vi "JKISM++ State Dashboard - DebugTool.vi"() -> ()   [LabVIEW 2014]
uses:
  _Support/Typedef/_JKI StateMachine Current State.ctl
  <resource>/dialog/lvconfig.llb/LV Config Read String.vi
  <resource>/dialog/lvconfig.llb/LV Config Read Numeric (I32).vi
  <resource>/dialog/lvconfig.llb/LV Config Write Numeric (I32).vi
  _Support/GlobalEvent/FGV-GlobalEventRef.vi
  _Support/jkism-tool-support.lvlib
  JKI-State-Machine-Plus.lvlib
panel:
  out "Dashboard":T1(array[cluster])
  out "State History":string
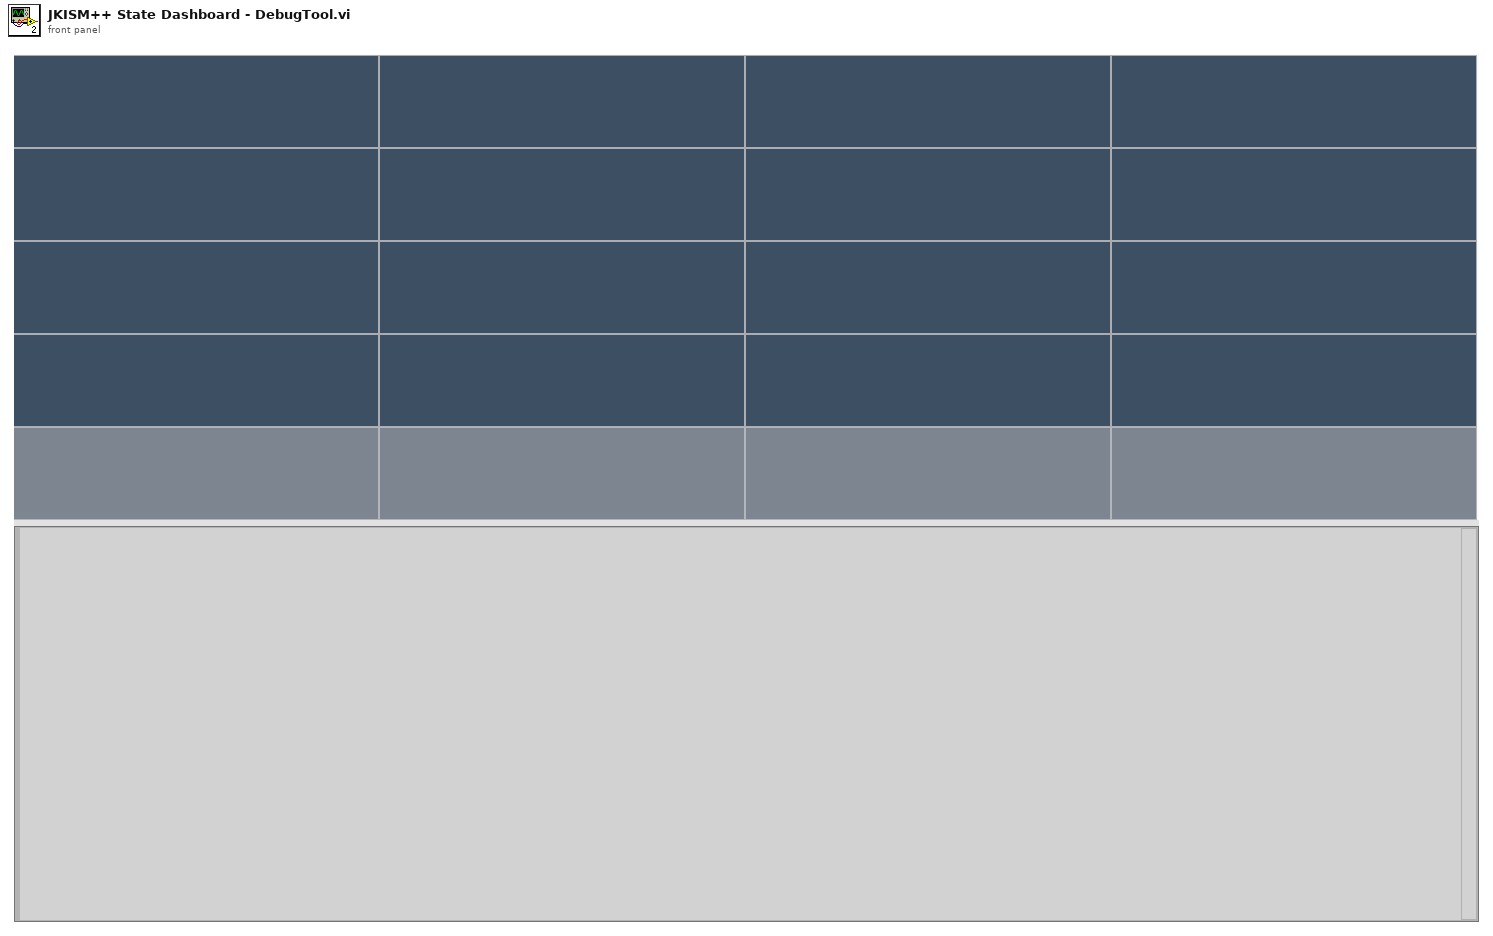
[diagram p1: front panel]
types:
  T1 = cluster{"Label":string, "Value":string, "String":string}[][]
  T2 = typedef "JKI-State-Machine-Plus.lvlib/_JKI StateMachine Current State.ctl" = cluster{"Name(\"\" to use uuid)":string, "Current State":string, "Arguments":string, "Argument - State":string, "From Who":string}
  T3 = enum32{"Invalid", "Standard", "Closed", "Hidden", "Minimized", "Maximized"}
  T4 = enum32{"invalid app kind", "Development System", "Run Time System", "Student Edition", "Embedded LabVIEW", "Evaluation", "Custom"}
  T5 = cluster{"Label":string, "Value":string, "String":string}
  T6 = cluster{"Core":cluster{"Current VI Reference":refnum<vi>, "Close Panel on Exit?":bool}, "Global-DataTable":string[][], "NumCols":i16, "NumRows":i16, "ApplicationName":string, "JKISM Global Log Event":refnum<user-event>}
  T7 = cluster{"Current VI Reference":refnum<vi>, "Close Panel on Exit?":bool}
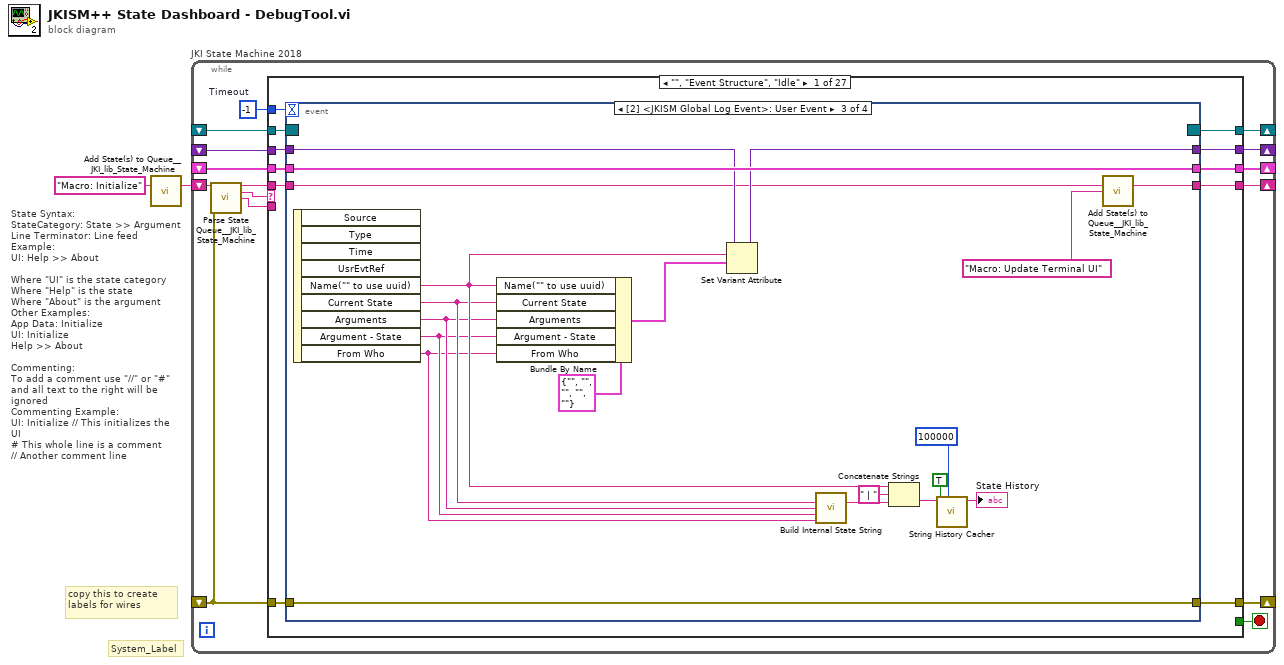
[diagram p0: block diagram]
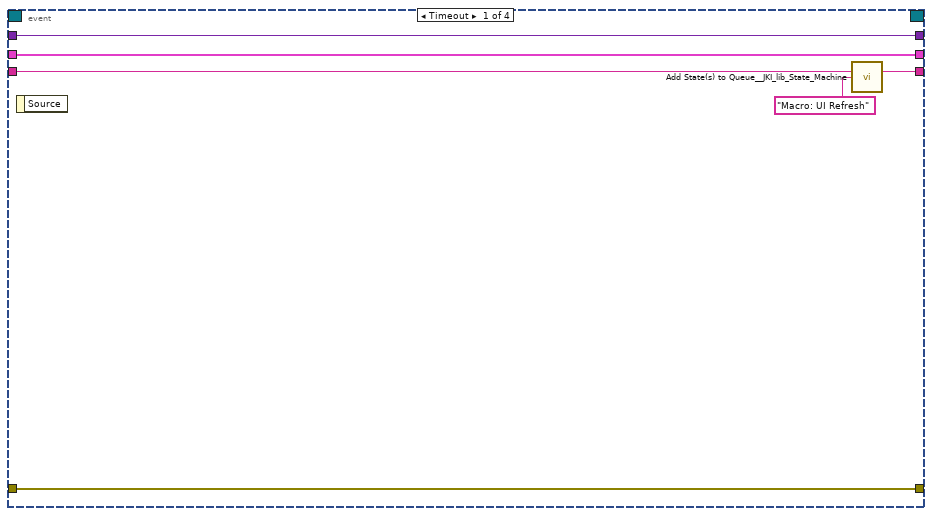
[diagram p2: hidden frame]
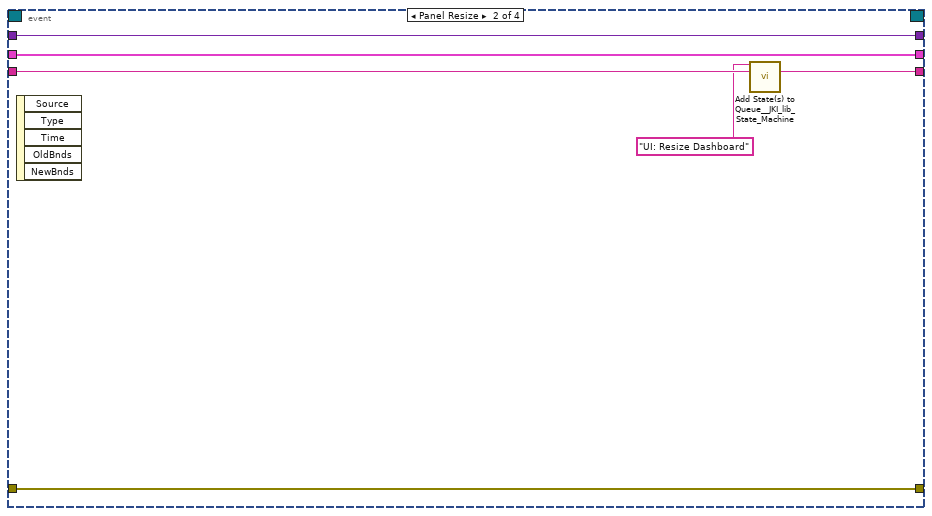
[diagram p3: hidden frame]
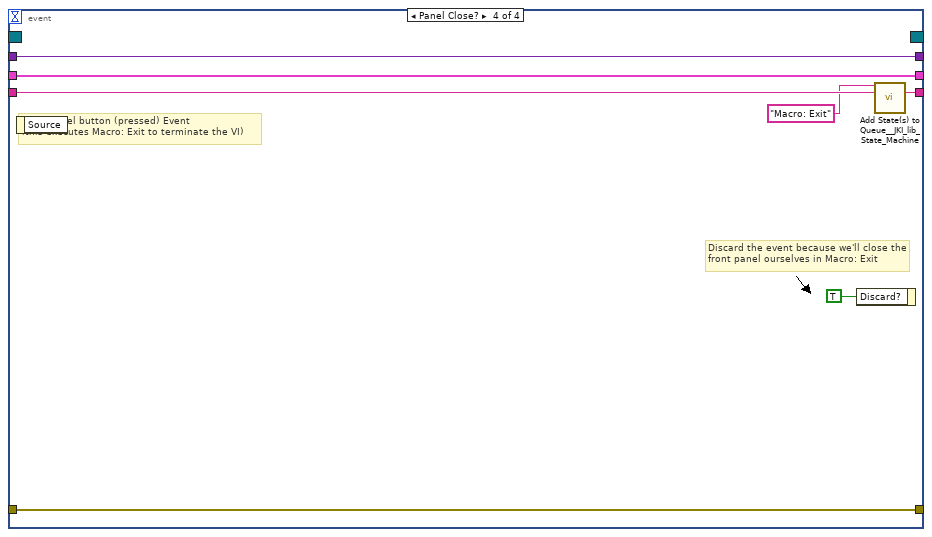
[diagram p4: hidden frame]
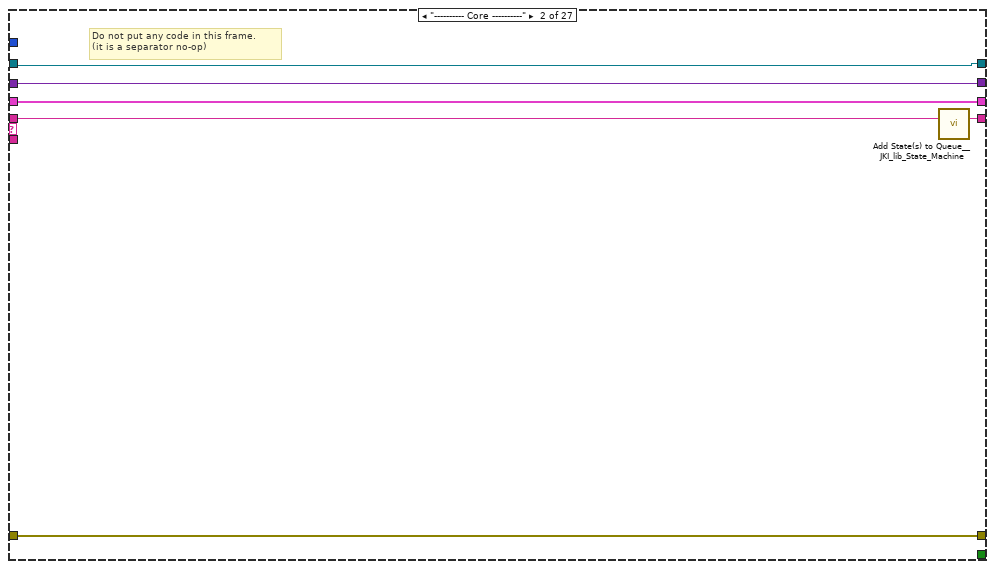
[diagram p5: hidden frame]
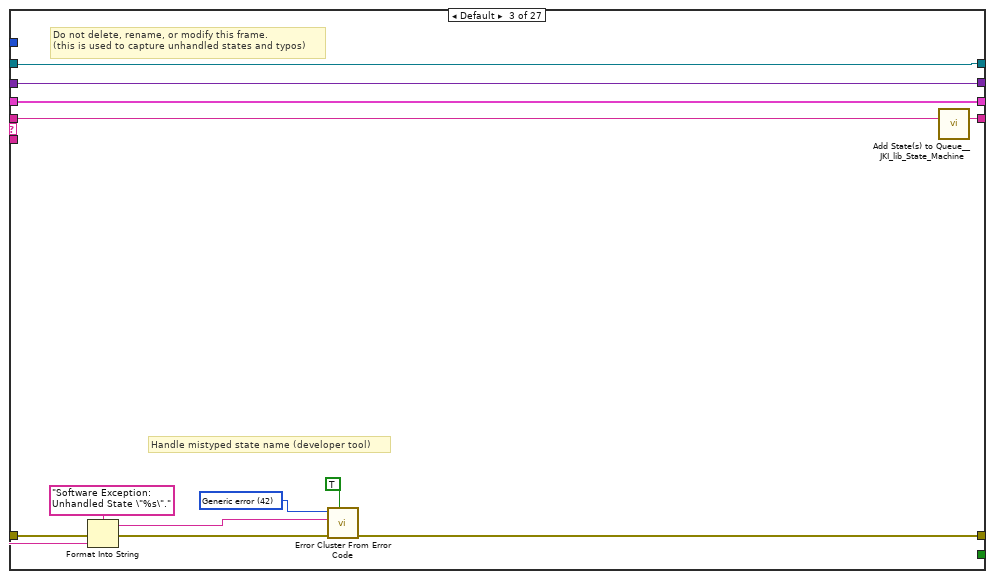
[diagram p6: hidden frame]
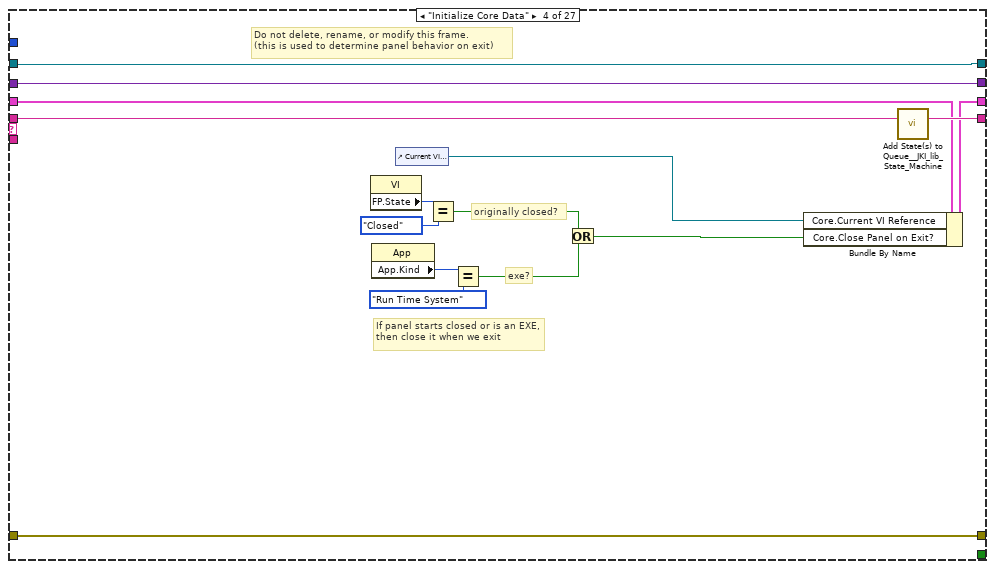
[diagram p7: hidden frame]
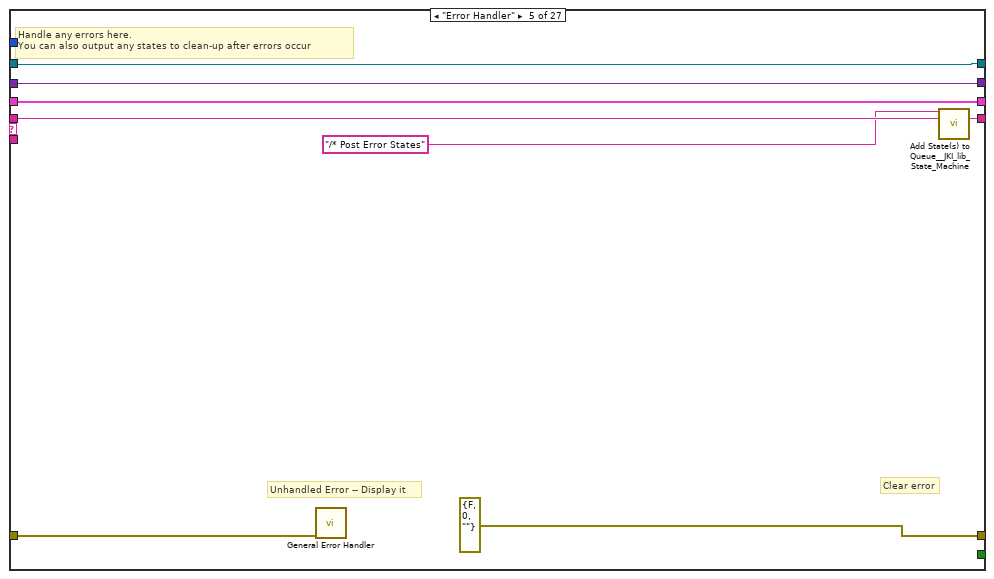
[diagram p8: hidden frame]
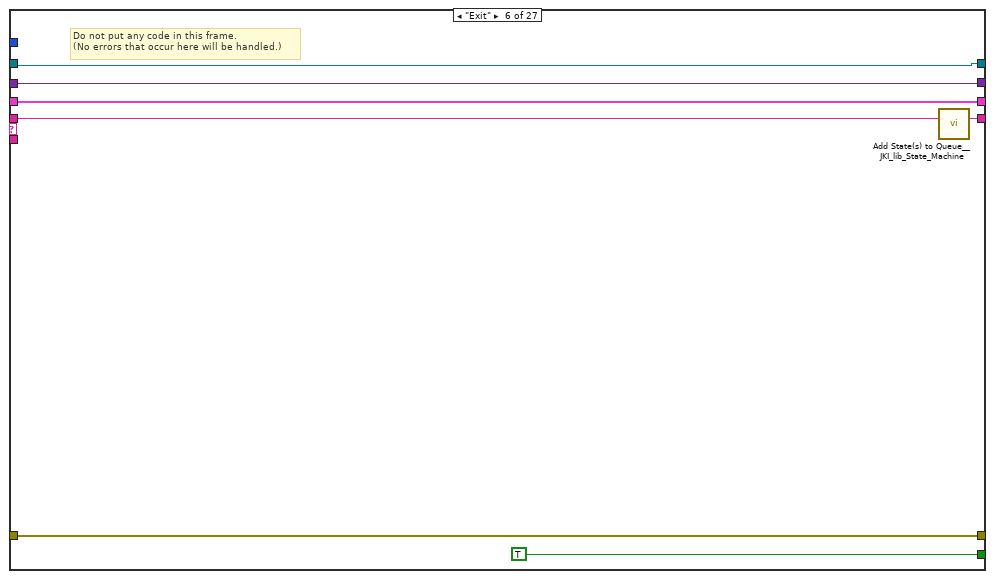
[diagram p9: hidden frame]
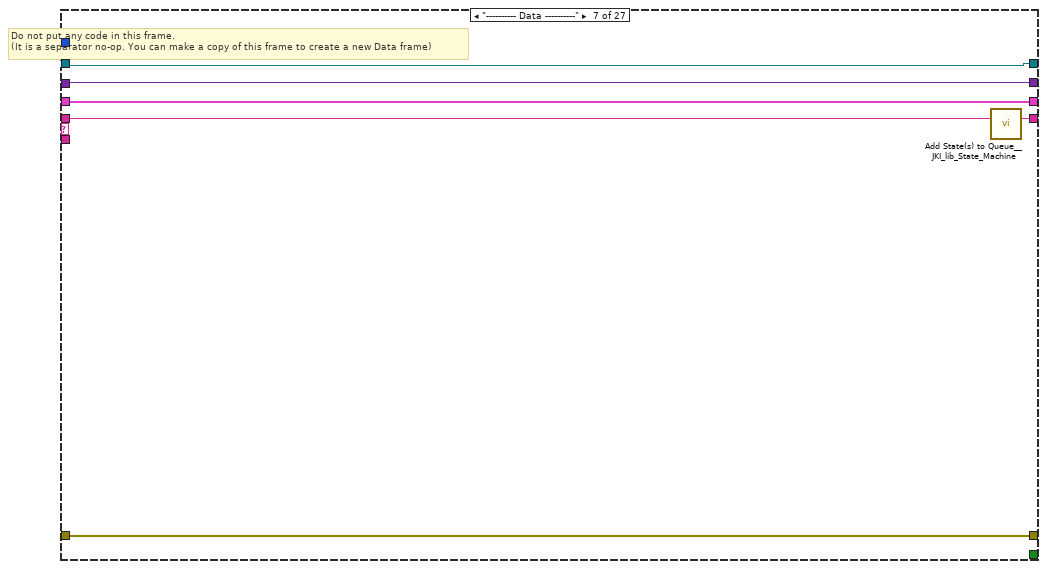
[diagram p10: hidden frame]
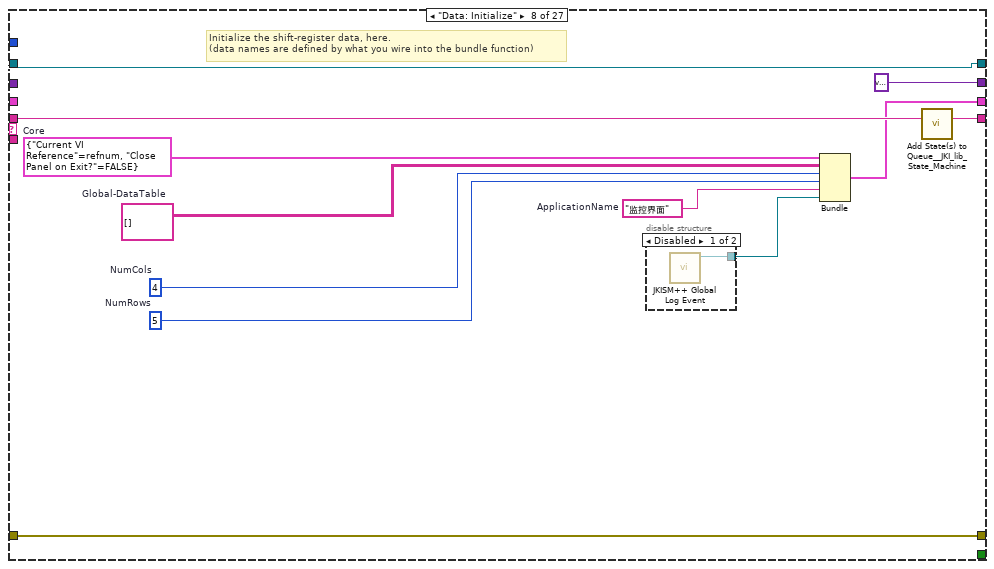
[diagram p11: hidden frame]
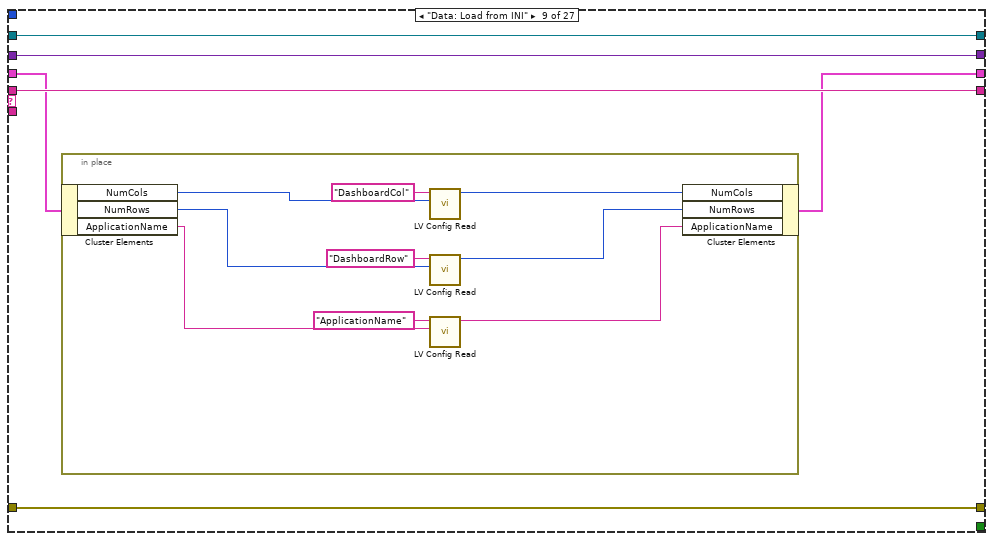
[diagram p13: hidden frame]
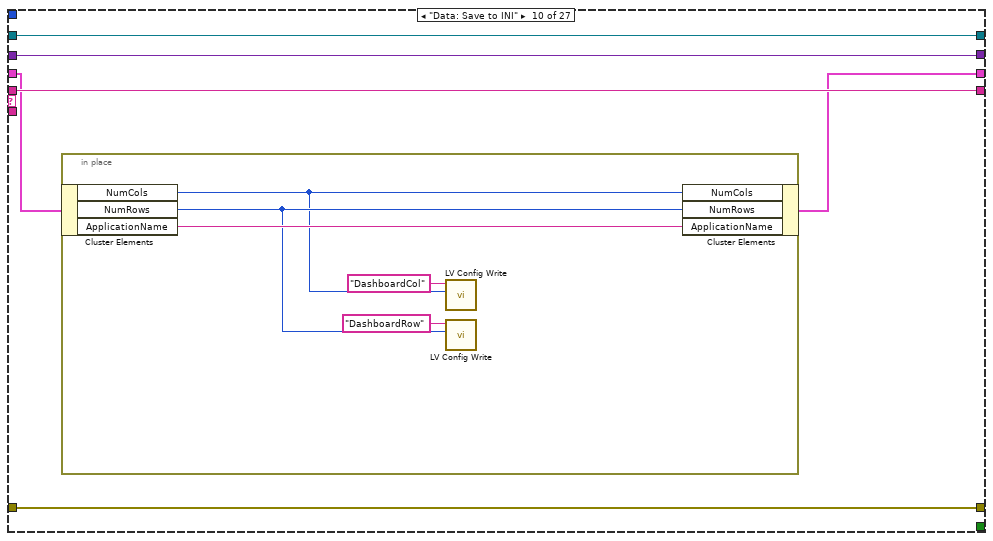
[diagram p14: hidden frame]
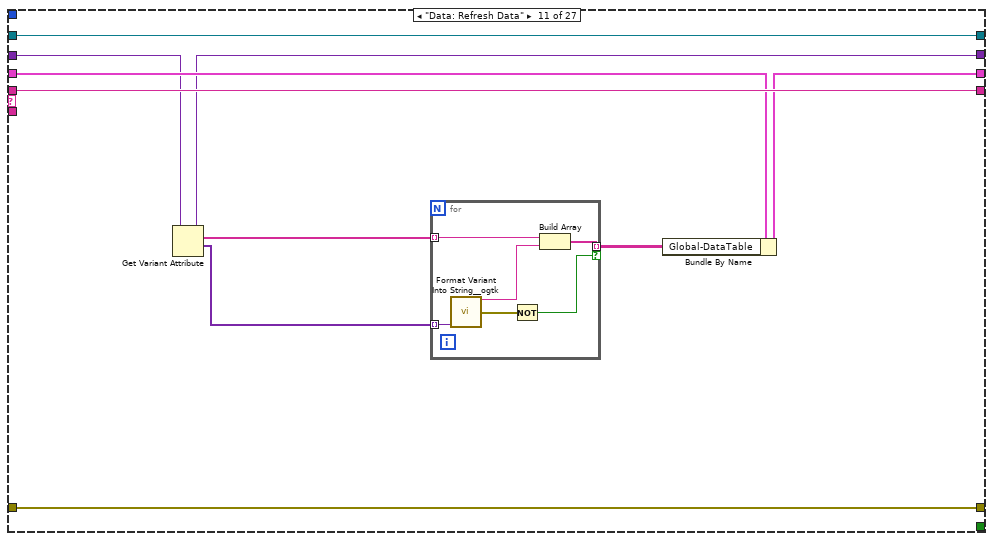
[diagram p15: hidden frame]
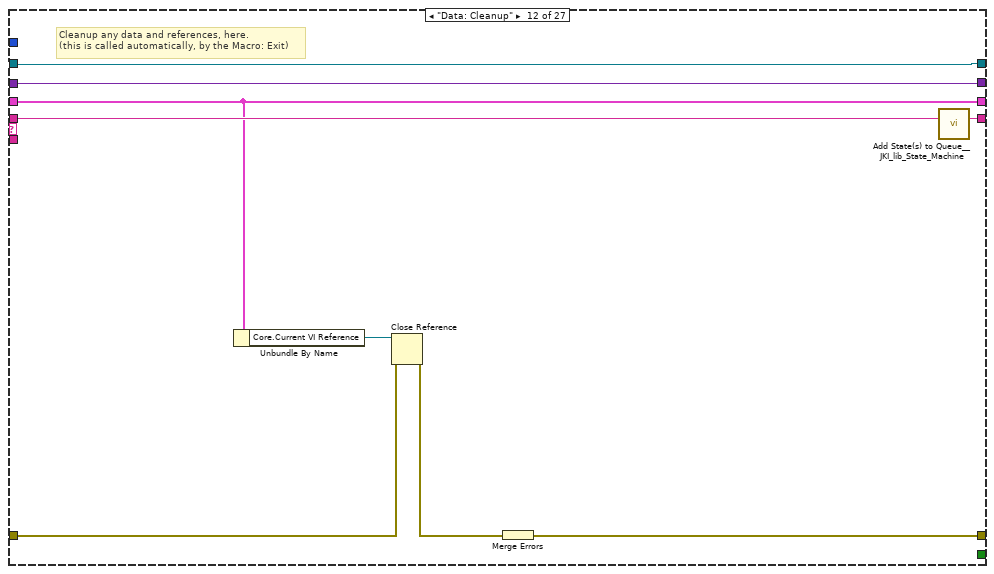
[diagram p16: hidden frame]
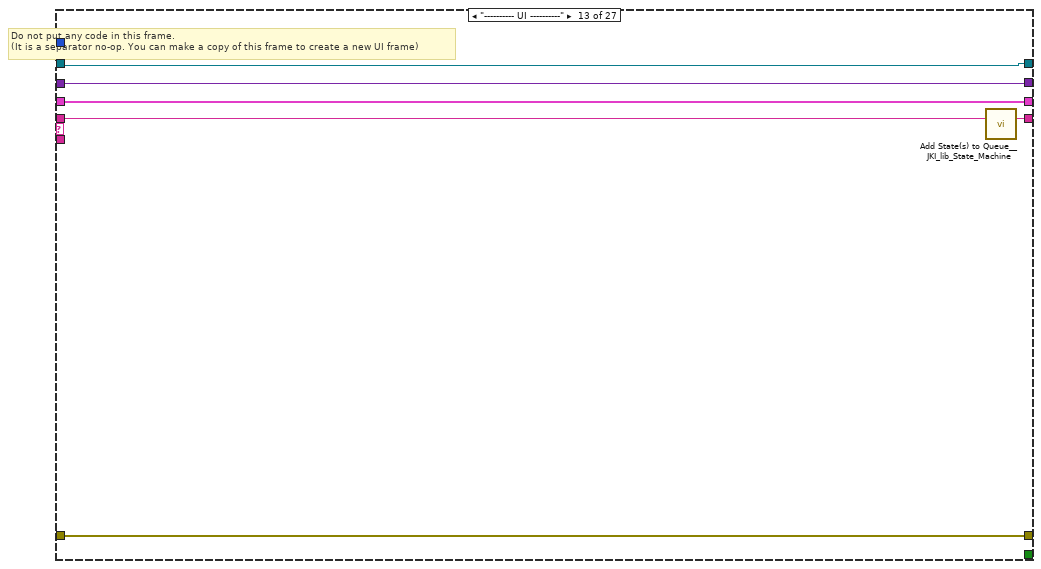
[diagram p17: hidden frame]
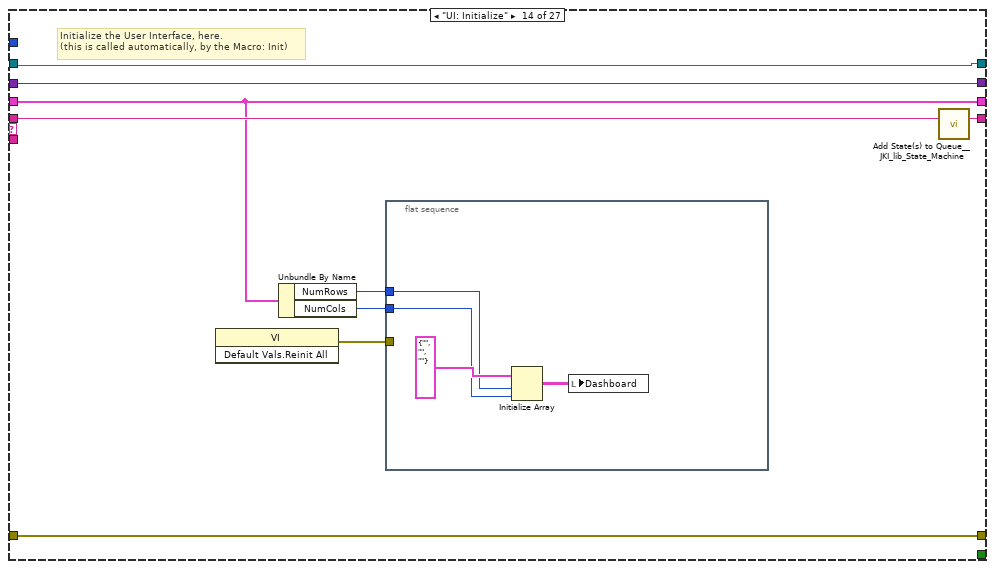
[diagram p18: hidden frame]
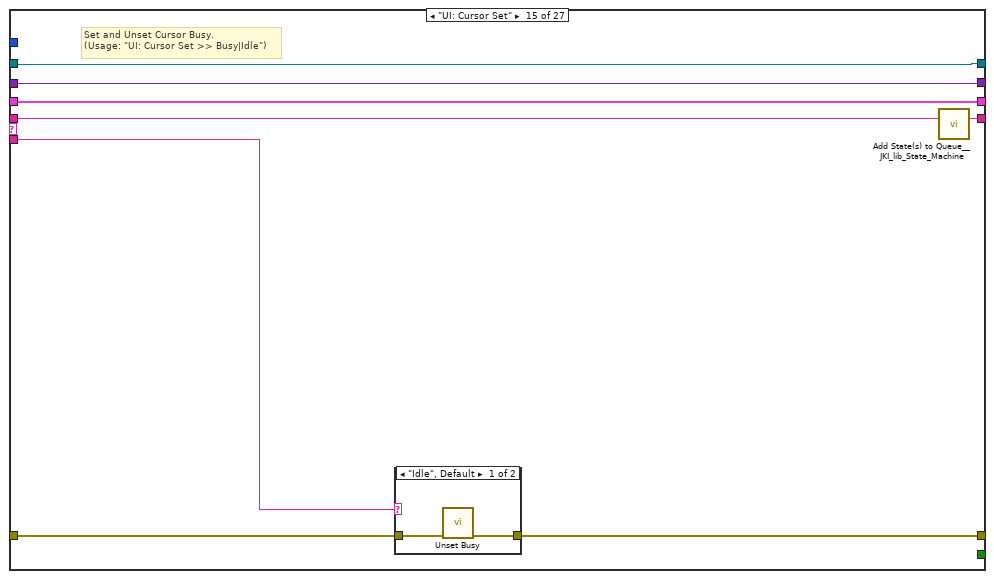
[diagram p19: hidden frame]
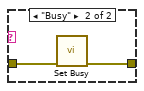
[diagram p20: hidden frame]
diagram:
  # "State Syntax:\nStateCategory: State >> Argument\nLine Terminator: Line feed\nExample:\nUI: Help >> About\n\nWhere \"UI\" is the state category\nWhere \"Help\" is the state\nWhere \"About\" is the argument\nOther Examples:\nApp Data: Initialize\nUI: Initialize\nHelp >> About\n\nCommenting:\nTo add a comment use \"//\" or \"#\" and all text to the right will be ignored\nCommenting Example:\nUI: Initialize // This initializes the UI\n# This whole line is a comment\n// Another comment line"
  # "copy this to create labels for wires"
  # "System_Label"
  n1 = call <vilib>:"Add State(s) to Queue__JKI_lib_State_Machine.vi"("State(s) in (\"\")"="Macro: Initialize") -> ("States Out"=w1:string)  [unwired: 14 in]
  n2 = while "JKI State Machine 2018" {
    shift-right: [w10] -> _
    shift-left: _ -> [w9]
    shift-right: [w13] -> _
    shift-left: _ -> [w7]
    shift-right: [w12] -> _
    shift-left: w1 -> [w14]
    shift-right: [w6] -> _
    shift-left: _ -> [w5]
    shift-right: [w4] -> _
    shift-left: _ -> [w3]
    stop <- w11 stop-if-true
    w8 = -1  # Timeout
    n3 = call <vilib>:"Parse State Queue__JKI_lib_State_Machine.vi"("State Queue"=w14, "Error In (no error)"=w7) -> ("Remaining States"=w16:string, "Current State"=w17:string, "Arguments"=w15:string)  [unwired: 11 in]
    n4 = case shown="\"\", \"Event Structure\", \"Idle\"" w17 {
      selector: w17 -> [_ _ w76 _ _ _ _ _ _ _ _ _ _ _ _ _ _ _ _ _ _ _ _ _ _ _ _]
      tunnel: w16 -> [w28 w73 w80 w101 w109 w116 w122 w134 w140 w155 w170 w186 w192 w201 w213 w226 w302 w309 w324 w334 w342 w350 w357 w364 w373 w380 w393]
      tunnel: w15 -> [_ _ _ _ _ _ _ _ _ _ _ _ _ _ w208 w220 _ _ _ _ _ _ _ _ _ _ _]
      tunnel: w9 -> [w26 w70 w78 w94 w106 w114 w119 _ w139 w154 w169 w181 w189 w197 w211 w222 w298 w306 w321 w333 w341 w346 w354 w361 w367 w377 w390]
      tunnel: [w25 w71 w82 w98 errorcluster {"status"=FALSE, "code"=0, "source"=""} ("error out") w113 w120 w130 w141 w156 w171 w180 w190 w199 w209 w223 w299 w307 w322 w335 w343 w351 w355 w362 w371 w378 w391] -> w13
      tunnel: w7 -> [w24 w71 w81 w98 w105 w113 w120 w130 w141 w156 w171 w183 w190 w199 w210 w224 _ w307 w322 w335 w343 w351 w355 w362 w371 w378 w391]
      tunnel: [w27 w72 w79 w100 w108 w115 w121 w133 w140 w155 w170 w185 w191 w200 w212 w225 w301 w308 w323 w334 w342 w350 w356 w363 w372 w379 w392] -> w12
      tunnel: [_ _ _ _ _ TRUE _ _ _ _ _ _ _ _ _ _ _ _ _ _ _ _ _ _ _ _ _] -> w11
      tunnel: [w23 w70 w78 w99 w106 w114 w119 w132 w138 w153 w168 w181 w189 w197 w211 w222 w298 w306 w321 w333 w337 w346 w354 w361 w367 w377 w390] -> w10
      tunnel: w8 -> [w22 _ _ _ _ _ _ _ _ _ _ _ _ _ _ _ _ _ _ _ _ _ _ _ _ _ _]
      tunnel: [w20 w69 w75 w88 w103 w111 w118 variant w137 w152 w165 w179 w188 w194 w207 w219 w295 w304 w316 w332 w340 w349 w353 w359 w366 w375 w383] -> w6
      tunnel: w5 -> [w21 w69 w75 w88 w103 w111 w118 _ w137 w152 w166 w179 w188 w194 w207 w219 w295 w304 w315 w332 w340 w349 w353 w359 w366 w375 w383]
      tunnel: [w18 w68 w74 w87 w102 w110 w117 w124 w136 w151 w162 w178 w187 w193 w206 w218 w294 w303 w312 w331 w338 w348 w352 w358 w365 w374 w382] -> w4
      tunnel: w3 -> [w19 w68 w74 w87 w102 w110 w117 w124 w136 w151 w162 w178 w187 w193 w206 w218 w294 w303 w312 w331 _ w348 w352 w358 w365 w374 w382]
      frame "", "Event Structure", "Idle" {
        n5 = event shown="[2] <JKISM Global Log Event>: User Event" {
          selector: w19 -> [_ _ _ _]
          dyn-events: [_ _ _ _] -> w18
          timeout: w22 -> [_ _ _ _]
          tunnel: w28 -> [w34 w37 w53 w67]
          tunnel: [w33 w38 w54 w66] -> w27
          tunnel: w26 -> [w31 w39 w59 w65]
          tunnel: [w32 w40 w60 w62] -> w25
          tunnel: w24 -> [w32 w40 w60 w62]
          tunnel: [w31 w39 w59 w65] -> w23
          tunnel: w21 -> [w29 w35 w58 w61]
          tunnel: [w29 w35 w57 w61] -> w20
          event Timeout {
            n6 = event-data() -> ()  [unwired: 1 in, 1 out]
            n7 = call <vilib>:"Add State(s) to Queue__JKI_lib_State_Machine.vi"("State(s) in (\"\")"=w34, "State(s) at Back (\"\")"="Macro: UI Refresh" ("State(s) in Front (\"\")")) -> ("States Out"=w33:string)  [unwired: 13 in]
          }
          event Panel Resize {
            n8 = event-data() -> ()  [unwired: 1 in, 5 out]
            n9 = call <vilib>:"Add State(s) to Queue__JKI_lib_State_Machine.vi"("State(s) in Front (\"\")"="UI: Resize Dashboard" ("State(s) in Front (\"\")"), "State(s) in (\"\")"=w37) -> ("States Out"=w38:string)  [unwired: 13 in]
          }
          event User Event {
            n10 = event-data() -> ("Name(\"\" to use uuid)"=w45:string, "Current State"=w44:string, "Arguments"=w43:string, "Argument - State"=w42:string, "From Who"=w41:string)  [unwired: 1 in, 4 out]
            n11 = Bundle By Name(cluster=T2 {"Name(\"\" to use uuid)"="", "Current State"="", "Arguments"="", "Argument - State"="", "From Who"=""} ("Cross JKI State Machine Data"), "Name(\"\" to use uuid)"=w45, "Current State"=w44, "Arguments"=w43, "Argument - State"=w42, "From Who"=w41) -> (w55:T2)
            n12 = Set Variant Attribute(Variant=w58, name=w45, value=w55) -> (Variant out=w57:variant)  [unwired: 1 in, 2 out]
            n13 = call "Build Internal State String.vi"("State"=w44, "Arguments (\"\")"=w43, "Arg-State (\"\")"=w42, "Source (\"\")"=w41) -> ("State with Arguments"=w51:string)  [unwired: 11 in]
            n14 = Concatenate Strings(w45, " | " ("string"), w51) -> (w48:string)
            n15 = call "String History Cacher.vi"("length"=100000, "Include Timestamp(F)"=TRUE, "String"=w48) -> ("String Cache"=→"State History":string)  [unwired: 8 in]
            n16 = call <vilib>:"Add State(s) to Queue__JKI_lib_State_Machine.vi"("State(s) in (\"\")"=w53, "State(s) at Back (\"\")"="Macro: Update Terminal UI" ("State(s) at Back (\"\")")) -> ("States Out"=w54:string)  [unwired: 13 in]
          }
          event Panel Close? {
            # "Discard the event because we'll close the front panel ourselves in Macro: Exit"
            # "Close Panel button (pressed) Event\n(this executes Macro: Exit to terminate the VI)"
            n17 = event-data() -> ()  [unwired: 1 in, 1 out]
            n18 = event-data("Discard?"=TRUE) -> ()  [unwired: 1 in, 1 out]
            n19 = call <vilib>:"Add State(s) to Queue__JKI_lib_State_Machine.vi"("State(s) in Front (\"\")"="Macro: Exit", "State(s) in (\"\")"=w67) -> ("States Out"=w66:string)  [unwired: 13 in]
          }
        }
      }
      frame "---------- Core ----------" {
        # "Do not put any code in this frame.\n(it is a separator no-op)"
        n20 = call <vilib>:"Add State(s) to Queue__JKI_lib_State_Machine.vi"("State(s) in (\"\")"=w73) -> ("States Out"=w72:string)  [unwired: 14 in]
      }
      frame Default {
        w85 = 42 items=["No error", "Argument error", "Memory is full", "Out of zone", "End of file", "File already open", "Generic file I/O error", "File not found", "File permission error", "Disk is full", "Duplicate path", "Too many files open", "System feature not enabled", "Resource file not found", "Cannot add resource", "Resource not found", "Image not found", "Image memory error", "Pen does not exist", "Config type invalid", "Config token not found", "Config parse error", "Config memory error", "Bad external code format", "Bad external code offset", "External code not present", "Null window", "Destroy window error", "Null menu", "Print aborted", "Bad print record", "Print driver error", "Windows error during printing", "Memory error during printing", "Print dialog error", "Generic print error", "Invalid device refnum", "Device not found", "Device parameter error", "Device unit error", "Cannot open device", "Device call aborted", "Generic error", "Cancelled by user", "Object ID too low", "Object ID too high", "Object not in heap", "Unknown heap", "Unknown object (invalid DefProc)", "Unknown object (DefProc not in table)", "Message out of range", "Invalid (null) method", "Unknown message", "Manager call not supported", "Bad address", "Network operation in progress", "Network operation timed out", "Connection is busy", "Network attribute not supported", "Network error", "Address in use", "System out of memory", "Connection aborted", "Connection refused", "Not connected", "Already connected", "Connection closed", "Initialization error (interapplication manager)", "Bad occurrence", "Wait on unbound occurrence handler", "Occurrence queue overflow", "Datalog type conflict", "Unused", "Unrecognized type (interapplication manager)", "Memory corrupt", "Failed to make temporary DLL", "Old CIN version", "Drag socket not found", "Failed to load drop-object", "Failed to register OLE object", "Failed to release OLE object", "Format specifier type mismatch", "Unknown format specifier", "Too few format specifiers", "Too many format specifiers", "Scan failed", "Newer CIN version", "Error converting to variant", "Runtime menu error", "Password tampered", "Variant attribute not found", "Incompatible variant data type", "Event data is not available", "Event Store is not present", "Occurrence is not found", "Event Queue is not created", "Event info is not available", "Refnum passed is NULL", "Error retrieving Class GUID", "Error retrieving CoClass GUID", "Error retrieving TypeLib GUID.", "Bad built application magic bytes.", "Specific driver is different from the specific driver associated with the Logical Name.", "There is no session opened to the class driver.", "Max Error", "MAX - Error with config objects", "MAX - Error loading configuration", "MAX - Group not supported"]
        # "Current State"
        # "Do not delete, rename, or modify this frame.\n(this is used to capture unhandled states and typos)"
        # "Handle mistyped state name (developer tool)"
        n21 = Format Into String(format string="Software Exception: Unhandled State \"%s\"." ("message"), error in=w81, w76) -> (resulting string=w84:string, error out=w83:errorcluster)  [unwired: 1 in]
        n22 = call <vilib>:"Error Cluster From Error Code.vi"("show call chain? (False)"=TRUE, "error in (no error)"=w83, "error message (\"\")"=w84, "error code (0)"=w85) -> ("error out"=w82:errorcluster)  [unwired: 5 in]
        n23 = call <vilib>:"Add State(s) to Queue__JKI_lib_State_Machine.vi"("State(s) in (\"\")"=w80) -> ("States Out"=w79:string)  [unwired: 14 in]
      }
      frame "Initialize Core Data" {
        # "Do not delete, rename, or modify this frame.\n(this is used to determine panel behavior on exit)"
        # "originally closed?"
        # "exe?"
        # "If panel starts closed or is an EXE, then close it when we exit"
        n24 = property class="VI"() -> ("FP.State"=w91:T3)  [unwired: 2 in, 2 out]
        n25 = property class="App"() -> ("App.Kind"=w97:T4)  [unwired: 2 in, 2 out]
        n26 = control-ref of="Current VI Reference"() -> (w92:refnum<vi>)
        n27 = Equal?(x=w91, y=T3."Closed" ("Front Panel Window:State")) -> (x = y?=w89:bool)
        n28 = Equal?(x=w97, y=T4."Run Time System" ("Application:Kind")) -> (x = y?=w95:bool)
        n29 = Or(x=w89, y=w95) -> (x .or. y?=w93:bool)
        n30 = Bundle By Name(cluster=w94, "Core.Current VI Reference"=w92, "Core.Close Panel on Exit?"=w93) -> (w99:T6)
        n31 = call <vilib>:"Add State(s) to Queue__JKI_lib_State_Machine.vi"("State(s) in (\"\")"=w101) -> ("States Out"=w100:string)  [unwired: 14 in]
      }
      frame "Error Handler" {
        # "Unhandled Error -- Display it"
        # "Handle any errors here.\nYou can also output any states to clean-up after errors occur"
        # "Clear error"
        n32 = call <vilib>:"General Error Handler.vi"("error in (no error)"=w105) -> ()  [unwired: 10 in, 5 out]
        n33 = call <vilib>:"Add State(s) to Queue__JKI_lib_State_Machine.vi"("State(s) in Front (\"\")"="/* Post Error States", "State(s) in (\"\")"=w109) -> ("States Out"=w108:string)  [unwired: 13 in]
      }
      frame "Exit" {
        # "Do not put any code in this frame.\n(No errors that occur here will be handled.)"
        n34 = call <vilib>:"Add State(s) to Queue__JKI_lib_State_Machine.vi"("State(s) in (\"\")"=w116) -> ("States Out"=w115:string)  [unwired: 14 in]
      }
      frame "---------- Data ----------" {
        # "Do not put any code in this frame.\n(It is a separator no-op. You can make a copy of this frame to create a new Data frame)"
        n35 = call <vilib>:"Add State(s) to Queue__JKI_lib_State_Machine.vi"("State(s) in (\"\")"=w122) -> ("States Out"=w121:string)  [unwired: 14 in]
      }
      frame "Data: Initialize" {
        w126 = "监控界面"  # ApplicationName
        w128 = i16 4  # NumCols
        w127 = i16 5  # NumRows
        w129 = string[][] []  # Global-DataTable
        w131 = T7 {"Current VI Reference"=refnum, "Close Panel on Exit?"=FALSE}  # Core
        # "Initialize the shift-register data, here.\n(data names are defined by what you wire into the bundle function)"
        n36 = disable-structure shown="Disabled" {
          disable-tunnel: [w135 _] -> w123
          frame Disabled {
            n37 = call "JKISM++ Global Log Event.vi"() -> ("JKISM Global Log Event"=w135:refnum<user-event>)  [unwired: 10 in, 1 out]
          }
          frame Enabled {
          }
        }
        n38 = Bundle("Core"=w131, "Global-DataTable"=w129, "NumCols"=w128, "NumRows"=w127, "ApplicationName"=w126, "JKISM Global Log Event"=w123) -> (w132:T6)  [unwired: 1 in]
        n39 = call <vilib>:"Add State(s) to Queue__JKI_lib_State_Machine.vi"("State(s) in (\"\")"=w134) -> ("States Out"=w133:string)  [unwired: 14 in]
      }
      frame "Data: Load from INI" {
        n40 = in-place {
          n41 = in-place-cluster #1(w139) -> ("NumCols"=w143:i16, "NumRows"=w146:i16, "ApplicationName"=w149:string)
          n42 = call-poly <resource>:"LV Config Read.vi"("default value"=w143, "key"="DashboardCol") -> ("value"=w142:i32)  [unwired: 3 in, 2 out]
          n43 = call-poly <resource>:"LV Config Read.vi"("default value"=w146, "key"="DashboardRow") -> ("value"=w145:i32)  [unwired: 3 in, 2 out]
          n44 = call-poly <resource>:"LV Config Read.vi"("default value"=w149, "key"="ApplicationName") -> ("value"=w148:string)  [unwired: 3 in, 2 out]
          n45 = in-place-cluster #1("NumCols"=w142, "NumRows"=w145, "ApplicationName"=w148) -> (w138:T6)
        }
      }
      frame "Data: Save to INI" {
        n46 = in-place {
          n47 = in-place-cluster #2(w154) -> ("NumCols"=w157:i16, "NumRows"=w158:i16, "ApplicationName"=w159:string)
          n48 = call-poly <resource>:"LV Config Write.vi"("value"=w157, "key"="DashboardCol") -> ()  [unwired: 5 in, 1 out]
          n49 = call-poly <resource>:"LV Config Write.vi"("value"=w158, "key"="DashboardRow") -> ()  [unwired: 5 in, 1 out]
          n50 = in-place-cluster #2("NumCols"=w157, "NumRows"=w158, "ApplicationName"=w159) -> (w153:T6)
        }
      }
      frame "Data: Refresh Data" {
        n51 = Get Variant Attribute(Variant=w166) -> (duplicate Variant=w165:variant, names=w164:string[], values=w163:variant[])  [unwired: 3 in, 1 out]
        n52 = for {
          tunnel: w163 -> [w177] mode=indexing
          tunnel: w164 -> [w176] mode=indexing
          tunnel: [w174] -> w167 mode=indexing if=w172
          n53 = call <userlib>:"Format Variant Into String__ogtk.vi"("Variant"=w177) -> ("Output String"=w175:string, "error out"=w173:errorcluster)  [unwired: 13 in]
          n54 = Not(x=w173) -> (.not. x?=w172:bool)
          n55 = Build Array(w176, w175) -> (w174:string[])
        }
        n56 = Bundle By Name(cluster=w169, "Global-DataTable"=w167) -> (w168:T6)
      }
      frame "Data: Cleanup" {
        # "Cleanup any data and references, here.\n(this is called automatically, by the Macro: Exit)"
        n57 = Unbundle By Name(w181) -> ("Core.Current VI Reference"=w184:refnum<vi>)
        n58 = Close Reference(reference=w184, error in (no error)=w183) -> (error out=w182:errorcluster)
        n59 = Merge Errors(w182) -> (w180:errorcluster)
        n60 = call <vilib>:"Add State(s) to Queue__JKI_lib_State_Machine.vi"("State(s) in (\"\")"=w186) -> ("States Out"=w185:string)  [unwired: 14 in]
      }
      frame "---------- UI ----------" {
        # "Do not put any code in this frame.\n(It is a separator no-op. You can make a copy of this frame to create a new UI frame)"
        n61 = call <vilib>:"Add State(s) to Queue__JKI_lib_State_Machine.vi"("State(s) in (\"\")"=w192) -> ("States Out"=w191:string)  [unwired: 14 in]
      }
      frame "UI: Initialize" {
        # "Initialize the User Interface, here.\n(this is called automatically, by the Macro: Init)"
        n62 = invoke class="VI" method="Default Vals.Reinit All"() -> (error out=w198:errorcluster)  [unwired: 3 in, 2 out]
        n63 = Unbundle By Name(w197) -> ("NumRows"=w196:i16, "NumCols"=w195:i16)
        n64 = flat-sequence {
          tunnel: w198 -> [_]
          tunnel: w196 -> [w203]
          tunnel: w195 -> [w202]
          frame #0 {
            n65 = Initialize Array(T5 {"Label"="", "Value"="", "String"=""} ("Dashboard"), w203, w202) -> (w204:T1)
            n66 = local write "Dashboard"(w204) -> ()
          }
        }
        n67 = call <vilib>:"Add State(s) to Queue__JKI_lib_State_Machine.vi"("State(s) in (\"\")"=w201) -> ("States Out"=w200:string)  [unwired: 14 in]
      }
      frame "UI: Cursor Set" {
        # "Argument"
        # "Set and Unset Cursor Busy.\n(Usage: \"UI: Cursor Set >> Busy|Idle\")"
        n68 = case shown="\"Idle\", Default" w208 {
          tunnel: w210 -> [w215 w217]
          tunnel: [w214 w216] -> w209
          frame "Idle", Default {
            n69 = call <vilib>:"Unset Busy.vi"("error in (no error)"=w215) -> ("error out"=w214:errorcluster)  [unwired: 10 in]
          }
          frame "Busy" {
            n70 = call <vilib>:"Set Busy.vi"("error in (no error)"=w217) -> ("error out"=w216:errorcluster)  [unwired: 9 in, 1 out]
          }
        }
        n71 = call <vilib>:"Add State(s) to Queue__JKI_lib_State_Machine.vi"("State(s) in (\"\")"=w213) -> ("States Out"=w212:string)  [unwired: 14 in]
      }
      frame "UI: Front Panel State" {
        # "Argument"
        # "Set Front Panel Open or Closed\n(Usage: \"UI: Front Panel State >> Open|Close\")"
        n72 = Unbundle By Name(w222) -> ("Core.Current VI Reference"=w221:refnum<vi>)
        n73 = case shown="\"Minimize\", \"Minimized\"" w220 {
          tunnel: w224 -> [w232 w247 w258 w271 w284]
          tunnel: [w234 w248 w260 w273 w286] -> w223
          tunnel: w221 -> [w233 w245 w259 w272 w285]
          frame "Open", "Standard", Default {
            w227 = T3."Standard" ("State")
            n74 = property class="VI"(reference=w233, error in=w232) -> (reference out=w230:refnum<vi>, error out=w231:errorcluster, "FP.State"=w229:T3)
            n75 = Not Equal?(x=w229, y=w227) -> (x != y?=w228:bool)
            n76 = case shown="True" w228 {
              tunnel: [w238 w240] -> w234
              tunnel: w231 -> [w237 w240]
              tunnel: w230 -> [w236 _]
              tunnel: w227 -> [w235 _]
              frame True {
                n77 = invoke class="VI" method="FP.Open"(reference=w236, error in=w237, "Activate"=TRUE, "State"=w235) -> (error out=w238:errorcluster)  [unwired: 1 in, 4 out]
              }
              frame False {
              }
            }
          }
          frame "Close", "Closed" {
            n78 = property class="VI"(reference=w245, error in=w247) -> (reference out=w244:refnum<vi>, error out=w246:errorcluster, "FP.State"=w242:T3)
            n79 = Not Equal?(x=w242, y=T3."Closed" ("Front Panel Window:State")) -> (x != y?=w241:bool)
            n80 = case shown="True" w241 {
              tunnel: [w249 w252] -> w248
              tunnel: w246 -> [w249 w251]
              tunnel: w244 -> [_ w250]
              frame False {
              }
              frame True {
                n81 = invoke class="VI" method="FP.Close"(reference=w250, error in=w251) -> (error out=w252:errorcluster)  [unwired: 1 in, 2 out]
              }
            }
          }
          frame "Hidden", "Hide" {
            w253 = T3."Hidden" ("State")
            n82 = property class="VI"(reference=w259, error in=w258) -> (reference out=w256:refnum<vi>, error out=w257:errorcluster, "FP.State"=w255:T3)
            n83 = Not Equal?(x=w255, y=w253) -> (x != y?=w254:bool)
            n84 = case shown="True" w254 {
              tunnel: [w264 w265] -> w260
              tunnel: w257 -> [w263 w265]
              tunnel: w256 -> [w262 _]
              tunnel: w253 -> [w261 _]
              frame True {
                n85 = invoke class="VI" method="FP.Open"(reference=w262, error in=w263, "State"=w261) -> (error out=w264:errorcluster)  [unwired: 2 in, 4 out]
              }
              frame False {
              }
            }
          }
          frame "Minimize", "Minimized" {
            w266 = T3."Minimized" ("State")
            n86 = property class="VI"(reference=w272, error in=w271) -> (reference out=w269:refnum<vi>, error out=w270:errorcluster, "FP.State"=w268:T3)
            n87 = Not Equal?(x=w268, y=w266) -> (x != y?=w267:bool)
            n88 = case shown="True" w267 {
              tunnel: [w277 w278] -> w273
              tunnel: w270 -> [w276 w278]
              tunnel: w269 -> [w275 _]
              tunnel: w266 -> [w274 _]
              frame True {
                n89 = invoke class="VI" method="FP.Open"(reference=w275, error in=w276, "State"=w274) -> (error out=w277:errorcluster)  [unwired: 2 in, 4 out]
              }
              frame False {
              }
            }
          }
          frame "Maximize", "Maximized" {
            w279 = T3."Maximized" ("State")
            n90 = property class="VI"(reference=w285, error in=w284) -> (reference out=w282:refnum<vi>, error out=w283:errorcluster, "FP.State"=w281:T3)
            n91 = Not Equal?(x=w281, y=w279) -> (x != y?=w280:bool)
            n92 = case shown="True" w280 {
              tunnel: [w290 w291] -> w286
              tunnel: w283 -> [w289 w291]
              tunnel: w282 -> [w288 _]
              tunnel: w279 -> [w287 _]
              frame True {
                n93 = invoke class="VI" method="FP.Open"(reference=w288, error in=w289, "State"=w287) -> (error out=w290:errorcluster)  [unwired: 2 in, 4 out]
              }
              frame False {
              }
            }
          }
        }
        n94 = call <vilib>:"Add State(s) to Queue__JKI_lib_State_Machine.vi"("State(s) in (\"\")"=w226) -> ("States Out"=w225:string)  [unwired: 14 in]
      }
      frame "UI: Resize Dashboard" {
        # "Do not put any code in this frame.\n(It is a separator no-op. You can make a copy of this frame to create a new UI frame)"
        n95 = property on="Pane" class="Pane"() -> ("Width"=w292:u32, "Height"=w293:u32)  [unwired: 2 in, 2 out]
        n96 = control-ref of="Dashboard"() -> (w300:refnum<vi>)
        n97 = Unbundle By Name(w298) -> ("NumCols"=w296:i16, "NumRows"=w297:i16)
        n98 = call "DashboardCell2 Array Resize.vi"("NumCols"=w296, "NumRows"=w297, "area height"=w293, "area width"=w292, "Array 2"=w300) -> ("error out"=w299:errorcluster)  [unwired: 6 in]
        n99 = call <vilib>:"Add State(s) to Queue__JKI_lib_State_Machine.vi"("State(s) in (\"\")"=w302) -> ("States Out"=w301:string)  [unwired: 14 in]
      }
      frame "UI: Update Title" {
        # "Do not put any code in this frame.\n(It is a separator no-op. You can make a copy of this frame to create a new UI frame)"
        n100 = Unbundle By Name(w306) -> ("ApplicationName"=w305:string)
        n101 = property class="VI"("Front Panel.Title"=w305) -> ()  [unwired: 2 in, 2 out]
        n102 = call <vilib>:"Add State(s) to Queue__JKI_lib_State_Machine.vi"("State(s) in (\"\")"=w309) -> ("States Out"=w308:string)  [unwired: 14 in]
      }
      frame "UI: Update Dashboard" {
        # "Do not put any code in this frame.\n(It is a separator no-op. You can make a copy of this frame to create a new UI frame)"
        n103 = Get Variant Attribute(Variant=w315) -> (duplicate Variant=w316:variant, names=w314:string[], values=w313:variant[])  [unwired: 3 in, 1 out]
        n104 = Variant To Data(type=T2[] [], Variant=w313) -> (data=w310:T2[])  [unwired: 1 in, 1 out]
        n105 = for {
          tunnel: w314 -> [w329] mode=indexing
          tunnel: [w328] -> w320 mode=indexing
          tunnel: w310 -> [w327] mode=indexing
          n106 = Unbundle By Name(w327) -> ("Current State"=w326:string, "Arguments"=w325:string)  [unwired: 1 out]
          n107 = Bundle By Name(cluster=T5 {"Label"="", "Value"="", "String"=""}, "Label"=w329, "Value"=w326, "String"=w325) -> (w328:T5)
        }
        n108 = Unbundle By Name(w321) -> ("NumRows"=w318:i16, "NumCols"=w317:i16)
        n109 = Reshape Array(w320, w318, w317) -> (→"Dashboard":T1)
        n110 = call <vilib>:"Add State(s) to Queue__JKI_lib_State_Machine.vi"("State(s) in (\"\")"=w324) -> ("States Out"=w323:string)  [unwired: 14 in]
      }
      frame "--------- Event ---------" {
      }
      frame "Register User Event" {
        n111 = call "JKISM++ Global Log Event.vi"() -> ("Error out"=w339:errorcluster, "JKISM Global Log Event"=w336:refnum<user-event>)  [unwired: 10 in]
        n112 = register-events(error in=w339, w336) -> (reference out=w338:refnum<event-registration>)  [unwired: 1 in, 1 out]
        n113 = Bundle By Name(cluster=w341, "JKISM Global Log Event"=w336) -> (w337:T6)
      }
      frame "UnRegister User Event" {
        n114 = Unregister For Events(event registration refnum=w348) -> (error out=w347:errorcluster)  [unwired: 1 in]
        n115 = Unbundle By Name(w346) -> ("JKISM Global Log Event"=w345:refnum<user-event>)
        n116 = Destroy User Event(user event=w345, error in=w347) -> (error out=w344:errorcluster)
        n117 = call <vilib>:"Clear Errors.vi"("error in (no error)"=w344) -> ()  [unwired: 6 in, 1 out]
      }
      frame "---------- Macro ----------" {
        # "Do not put any code in this frame.\n(It is a separator no-op. You can make a copy of this frame to create a new Macro frame)"
        n118 = call <vilib>:"Add State(s) to Queue__JKI_lib_State_Machine.vi"("State(s) in (\"\")"=w357) -> ("States Out"=w356:string)  [unwired: 14 in]
      }
      frame "Macro: Initialize" {
        # "Initialization Macro\n(This is called once, when the VI starts)"
        n119 = call <vilib>:"Add State(s) to Queue__JKI_lib_State_Machine.vi"("State(s) in Front (\"\")"="Data: Initialize\nInitialize Core Data\nData: Load from INI\nUI: Initialize\nUI: Update Title\nUI: Resize Dashboard\nRegister User Event\n//UI: Front Panel State >> Open", "State(s) in (\"\")"=w364) -> ("States Out"=w363:string)  [unwired: 13 in]
      }
      frame "Macro: UI Refresh" {
        # "Do not put any code in this frame.\n(It is a separator no-op. You can make a copy of this frame to create a new Macro frame)"
        n120 = call <vilib>:"Add State(s) to Queue__JKI_lib_State_Machine.vi"("State(s) in Front (\"\")"="Data: Refresh Data" ("State(s) in Front (\"\")"), "State(s) at Back (\"\")"="Macro: Update Terminal UI" ("State(s) in Front (\"\")")) -> ("States Out"=w369:string)  [unwired: 13 in]
        n121 = call <vilib>:"Add State(s) to Queue__JKI_lib_State_Machine.vi"("State(s) in Front (\"\")"=w369, "State(s) in (\"\")"=w373) -> ("States Out"=w372:string)  [unwired: 13 in]
      }
      frame "Macro: Update Terminal UI" {
        # "Do not put any code in this frame.\n(It is a separator no-op. You can make a copy of this frame to create a new Macro frame)"
        n122 = call <vilib>:"Add State(s) to Queue__JKI_lib_State_Machine.vi"("State(s) in Front (\"\")"="UI: Update Dashboard" ("State(s) in Front (\"\")"), "State(s) in (\"\")"=w380) -> ("States Out"=w379:string)  [unwired: 13 in]
      }
      frame "Macro: Exit" {
        # "Exit Macro\n(This is called once, when the VI exits)"
        n123 = Unbundle By Name(w390) -> ("Core.Close Panel on Exit?"=w389:bool)
        n124 = Select(t="UI: Front Panel State >> Close", s=w389, f="") -> (s? t:f=w385:string)
        n125 = call <vilib>:"Add State(s) to Queue__JKI_lib_State_Machine.vi"("State(s) in Front (\"\")"="UnRegister User Event" ("State(s) in Front (\"\")"), "State(s) in (\"\")"=w385, "State(s) at Back (\"\")"="Data: Save to INI\nData: Cleanup\nExit") -> ("States Out"=w388:string)  [unwired: 12 in]
        n126 = call <vilib>:"Add State(s) to Queue__JKI_lib_State_Machine.vi"("State(s) in Front (\"\")"=w388, "State(s) in (\"\")"=w393) -> ("States Out"=w392:string)  [unwired: 13 in]
      }
    }
  }
